vi "runningLoop.vi"(8 "error in (no error)":errorcluster, 11 "HWController in":refnum<class "HWController.lvclass">) -> (0 "error out":errorcluster, 2 "userStoped":bool, 3 "HWController out":refnum<class "HWController.lvclass">)   [LabVIEW 2011, in "Hardware.lvlib" / "HWControllers.lvlib" / "HWController.lvclass"]
uses:
  HWController.lvclass
  HWController.lvclass/HWController.ctl
  HWControllerEvents/HWControllerEvents.lvclass
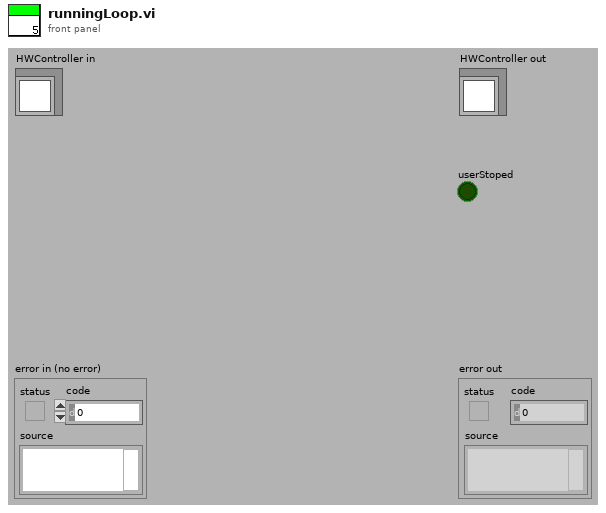
[diagram p1: front panel]
types:
  T1 = enum16{"Ready", "Compiling", "Configured", "Running", "Stopping", "Unresolved Error"}
  T2 = cluster{"incomingEventTypes":cluster{"start":cluster{"Boolean":bool}, "stop":cluster{"Boolean":bool}, "statusInquiry":cluster{"Boolean":bool}, "configure":cluster{"DPScriptPath":path, "TimeStamp":string, "HWLoop?":bool}, "resetError":cluster{"Boolean":bool}, "resourcesInquiry":cluster{"Boolean":bool}, "reserveResources":cluster{"HWList":string[]}, "initialise":cluster{"HWList":string[]}, "close":cluster{"Boolean":bool}, "resetAllChannels":cluster{"Boolean":bool}, "staticChannelUpdate":cluster{"channel_address":string, "calibratedValue":dbl}, "runScript":cluster{"DPScriptPath":path, "TimeStamp":string, "HWLoop?":bool}, "compilingScript":cluster{"Path":path}, "compiledScript":cluster{"Path":path, "timeCompileAt":string}, "compilerError":cluster{"Path":path}, "configureCompiledScript":cluster{"DPScriptPath":path, "TimeStamp":string, "HWLoop?":bool, "CompiledScript":cluster{"ScriptListCompiler.lvclass":refnum<class "ScriptListCompiler.lvclass">, "aoChannels":refnum<class "AnalogOutput.lvclass">[], "doChannels":refnum<class "DigitalOutput.lvclass">[], "rfChannels":refnum<class "DDSOutput.lvclass">[]}}, "restartCompiler":cluster{"restart":bool}, "staticRfChannelUpdate":cluster{"channel_address":string, "Output":cluster{"Frequency(MHz)":dbl, "Amplitude":dbl, "Phase":dbl, "OutputForm":enum16{"Sine", "Square", "Triangle", "Arbitrary"}}}, "cameraUpdate":cluster{"Camera":string, "Type":string, "settings":path}}, "outgoingEventTypes":cluster{"HWStatus":cluster{"status":enum16{"Ready", "Compiling", "Configured", "Running", "Stopping", "Unresolved Error"}}, "error":cluster{"error out":errorcluster}, "resourcesAvailable":cluster{"availableHWList":string[], "reservedHWList":string[]}, "resourcesReserved":cluster{"reservedHWList":string[]}}}
  T3 = enum16{"start", "stop", "statusInquiry", "configure", "resetError", "resourcesInquiry", "reserveResources", "initialise", "resetAllChannels", "staticUpdate", "close", "HWStatus", "error", "resourcesAvailable", "resourcesReserved", "compilerError", "compiledScript", "compilingScript", "runScript", "configureCompiledScript", "restartCompiler", "staticRfChannelUpdate", "cameraUpdate"}
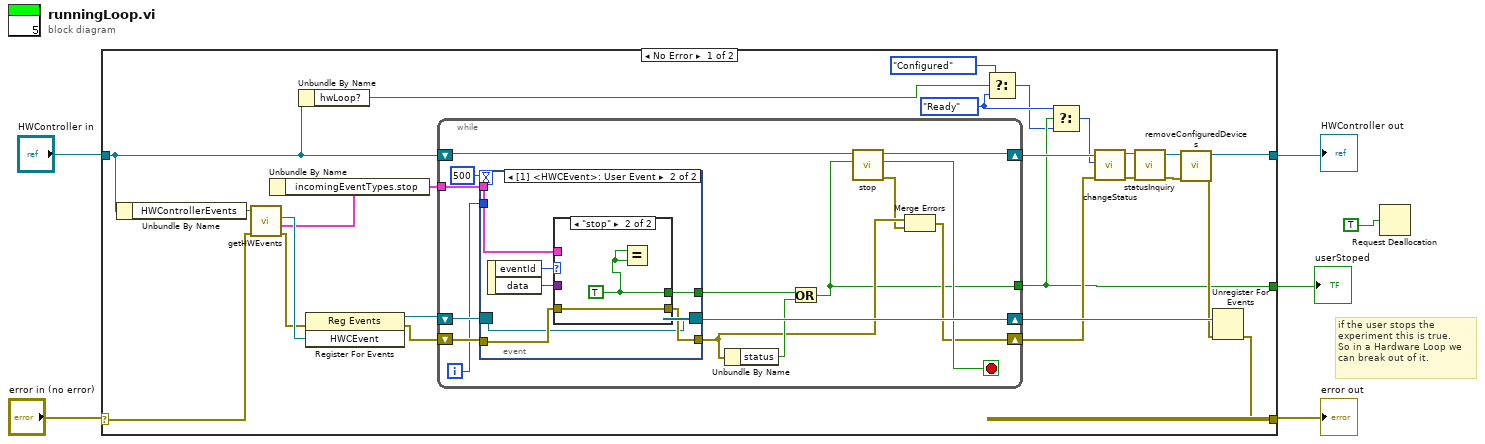
[diagram p0: block diagram]
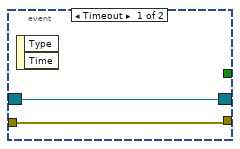
[diagram p2: hidden frame]
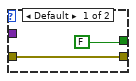
[diagram p3: hidden frame]
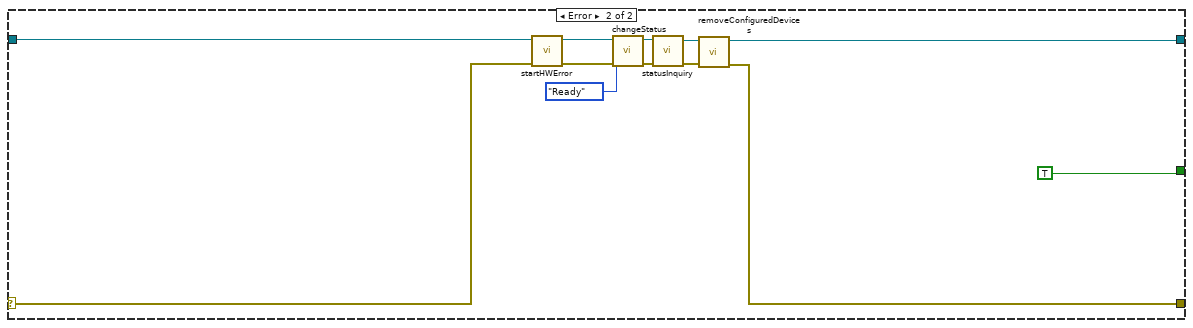
[diagram p4: hidden frame]
diagram:
  # "if the user stops the \nexperiment this is true.\nSo in a Hardware Loop we\ncan break out of it."
  n1 = case shown="No Error" "error in (no error)" {
    selector: "error in (no error)" -> [w30 w70]
    tunnel: [w24 w63] -> w5
    tunnel: [w16 w62] -> w3
    tunnel: "HWController in" -> [w13 w71]
    tunnel: [w9 TRUE] -> w1
    frame No Error {
      w8 = T1."Ready" ("status")
      n2 = Unbundle By Name(w13) -> ("HWControllerEvents"=w31:refnum<class "HWControllerEvents.lvclass">)
      n3 = call-dynamic "getHWEvents.vi"("error in (no error)"=w30, "HWControllerEvents in"=w31) -> ("error out"=w28:errorcluster, "eventDataTypes"=w19:T2, "HWCEvent"=w29:refnum<user-event>)  [unwired: 6 in, 1 out]
      n4 = Unbundle By Name(w19) -> ("incomingEventTypes.stop"=w18:cluster{"Boolean":bool})
      n5 = Unbundle By Name(w13) -> ("hwLoop?"=w12:bool)
      n6 = register-events(error in=w28, w29) -> (reference out=w27:refnum<event-registration>, error out=w26:errorcluster)  [unwired: 1 in]
      n7 = while {
        shift-right: [w45] -> w25
        shift-left: w27 -> [w46]
        shift-right: [w39] -> w22
        shift-left: w26 -> [w44]
        tunnel: w18 -> [w42]
        shift-right: [w32] -> w23
        shift-left: w13 -> [w33]
        tunnel: [w35] -> w9
        i -> [w37]
        stop <- w40 stop-if-true
        n8 = event shown="[1] <HWCEvent>: User Event" {
          selector: w46 -> [w48 w50]
          dyn-events: [w48 w50] -> w45
          timeout: 500 -> [_ _]
          tunnel: w44 -> [w47 w54]
          tunnel: [w47 w53] -> w38
          tunnel: w42 -> [_ w51]
          tunnel: w37 -> [_ _]
          tunnel: [_ w49] -> w36
          event Timeout {
            n9 = event-data() -> ()  [unwired: 1 in, 2 out]
          }
          event User Event {
            n10 = event-data() -> ("eventId"=w55:T3, "data"=w52:variant)  [unwired: 1 in]
            n11 = case shown="\"stop\"" w55 {
              tunnel: w52 -> [_ _]
              tunnel: w54 -> [w57 w59]
              tunnel: [w57 w59] -> w53
              tunnel: [FALSE w58] -> w49
              tunnel: w51 -> [_ _]
              frame Default {
              }
              frame "stop" {
                w58 = TRUE
                n12 = Equal?(x=w58, y=w58) -> ()  [unwired: 1 out]
              }
            }
          }
        }
        n13 = Unbundle By Name(w38) -> ("status"=w41:bool)
        n14 = Or(x=w36, y=w41) -> (x .or. y?=w35:bool)
        n15 = call-dynamic "stop.vi"("stop?"=w35, "HWController in"=w33) -> ("error out"=w34:errorcluster, "stopped"=w40:bool, "HWController out"=w32:refnum<class "HWController.lvclass">)  [unwired: 7 in]
        n16 = Merge Errors(w38, w34) -> (w39:errorcluster)
      }
      n17 = Select(t=T1."Configured" ("status"), s=w12, f=w8) -> (s? t:f=w7:T1)
      n18 = Select(t=w8, s=w9, f=w7) -> (s? t:f=w10:T1)
      n19 = call "changeStatus.vi"("error in (no error)"=w22, "status"=w10, "HWController in"=w23) -> ("error out"=w20:errorcluster, "HWController out"=w21:refnum<class "HWController.lvclass">)  [unwired: 7 in]
      n20 = call-dynamic "statusInquiry.vi"("error in (no error)"=w20, "HWController in"=w21) -> ("error out"=w15:errorcluster, "HWController out"=w17:refnum<class "HWController.lvclass">)  [unwired: 8 in]
      n21 = call "removeConfiguredDevices.vi"("error in (no error)"=w15, "HWController in"=w17) -> ("error out"=w14:errorcluster, "HWController out"=w16:refnum<class "HWController.lvclass">)  [unwired: 8 in]
      n22 = Unregister For Events(event registration refnum=w25, error in=w14) -> (error out=w24:errorcluster)
    }
    frame Error {
      n23 = call-dynamic "startHWError.vi"("error in (no error)"=w70, "HWController in"=w71) -> ("error out"=w64:errorcluster, "HWController out"=w65:refnum<class "HWController.lvclass">)  [unwired: 7 in, 1 out]
      n24 = call "changeStatus.vi"("error in (no error)"=w64, "status"=T1."Ready", "HWController in"=w65) -> ("error out"=w68:errorcluster, "HWController out"=w69:refnum<class "HWController.lvclass">)  [unwired: 7 in]
      n25 = call-dynamic "statusInquiry.vi"("error in (no error)"=w68, "HWController in"=w69) -> ("error out"=w66:errorcluster, "HWController out"=w67:refnum<class "HWController.lvclass">)  [unwired: 8 in]
      n26 = call "removeConfiguredDevices.vi"("error in (no error)"=w66, "HWController in"=w67) -> ("error out"=w63:errorcluster, "HWController out"=w62:refnum<class "HWController.lvclass">)  [unwired: 8 in]
    }
  }
  "error out" <- w5
  "HWController out" <- w3
  "userStoped" <- w1
  n27 = Request Deallocation(TRUE) -> ()
